vi "hw3.3.vi"() -> ()   [LabVIEW 2014]
panel:
  out "bubble":u32
  out "selection":u32
  out "insertion":u32
  out "selection Graph 3":dbl[](graph)
  out "insertion Graph 2":dbl[](graph)
  out "bubble Graph":dbl[](graph)
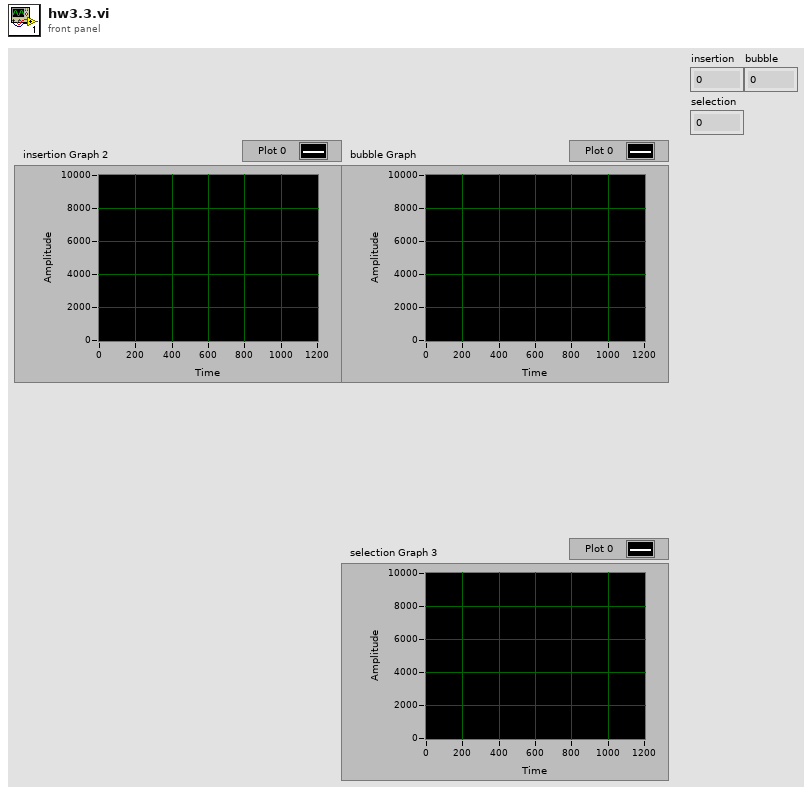
[diagram p1: front panel]
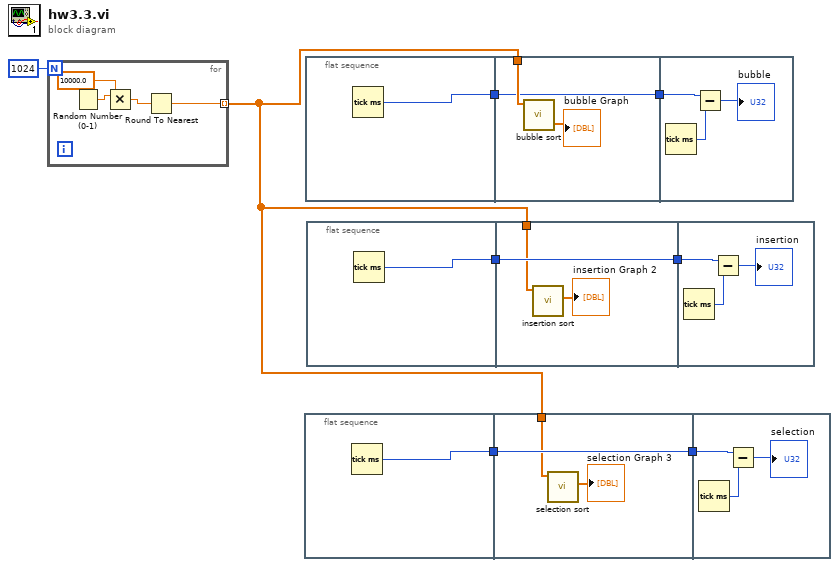
[diagram p0: block diagram]
diagram:
  n1 = for {
    N: 1024 -> [_]
    tunnel: [w9] -> w1 mode=indexing
    n2 = Random Number (0-1)() -> (number: 0 to 1=w12:dbl)
    n3 = Multiply(x=w12, y=10000.0) -> (x*y=w10:dbl)
    n4 = Round To Nearest(number=w10) -> (nearest integer value=w9:dbl)
  }
  n5 = flat-sequence {
    tunnel: [w13] -> w3
    tunnel: w3 -> [w16]
    tunnel: [w16] -> w2
    tunnel: w1 -> [w15]
    tunnel: w2 -> [w18]
    frame #0 {
      n6 = Tick Count (ms)() -> (millisecond timer value=w13:u32)
    }
    frame #1 {
      n7 = call "selection sort.vi"("Array in"=w15) -> ("Waveform Graph"=→"selection Graph 3":dbl[])  [unwired: 9 in, 1 out]
    }
    frame #2 {
      n8 = Tick Count (ms)() -> (millisecond timer value=w19:u32)
      n9 = Subtract(x=w18, y=w19) -> (x-y=→"selection":u32)
    }
  }
  n10 = flat-sequence {
    tunnel: [w20] -> w7
    tunnel: w1 -> [w23]
    tunnel: w7 -> [w21]
    tunnel: [w21] -> w6
    tunnel: w6 -> [w25]
    frame #0 {
      n11 = Tick Count (ms)() -> (millisecond timer value=w20:u32)
    }
    frame #1 {
      n12 = call "bubble sort.vi"("Array in"=w23) -> ("Waveform Graph"=→"bubble Graph":dbl[])  [unwired: 7 in, 3 out]
    }
    frame #2 {
      n13 = Tick Count (ms)() -> (millisecond timer value=w26:u32)
      n14 = Subtract(x=w25, y=w26) -> (x-y=→"bubble":u32)
    }
  }
  n15 = flat-sequence {
    tunnel: [w27] -> w5
    tunnel: w5 -> [w30]
    tunnel: [w30] -> w4
    tunnel: w1 -> [w29]
    tunnel: w4 -> [w32]
    frame #0 {
      n16 = Tick Count (ms)() -> (millisecond timer value=w27:u32)
    }
    frame #1 {
      n17 = call "insertion sort.vi"("Array in"=w29) -> ("Waveform Graph"=→"insertion Graph 2":dbl[])  [unwired: 9 in, 1 out]
    }
    frame #2 {
      n18 = Tick Count (ms)() -> (millisecond timer value=w33:u32)
      n19 = Subtract(x=w32, y=w33) -> (x-y=→"insertion":u32)
    }
  }
